vi "DQtoAlphaBeta_src.vi"(0 "direct":sgl format="%#_30g", 5 "quadrature":sgl format="%#_30g", 7 "theta":sgl) -> (4 "alpha":sgl format="%#_30g", 6 "beta":sgl format="%#_30g", 13 "sinx":sgl, 14 "cosx":sgl)   [LabVIEW 2015]
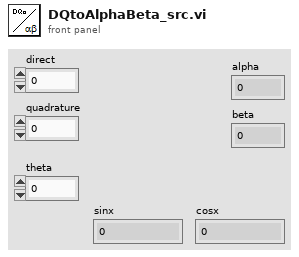
[diagram p1: front panel]
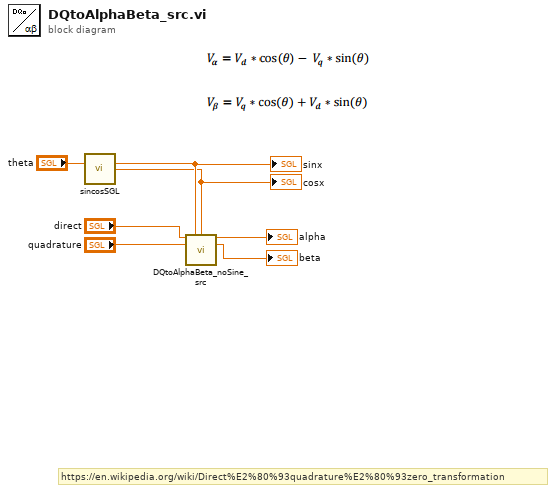
[diagram p0: block diagram]
diagram:
  # "https://en.wikipedia.org/wiki/Direct%E2%80%93quadrature%E2%80%93zero_transformation"
  n1 = call "sincosSGL.vi"("x"="theta") -> ("sinx"=w4:sgl, "cosx"=w3:sgl)  [unwired: 13 in]
  "sinx" <- w4
  "cosx" <- w3
  n2 = call "DQtoAlphaBeta_noSine_src.vi"("direct"="direct", "cosx"=w4, "sinx"=w3, "quadrature"="quadrature") -> ("alpha"=→"alpha":sgl, "beta"=→"beta":sgl)  [unwired: 10 in]
